vi "TCP Initialize Client.vi"   [LabVIEW 2016, in "SLL Easy API via TCP.lvclass"]
uses:
  SLL Easy API via TCP.lvclass
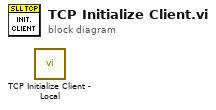
[diagram p0: block diagram]
diagram:
  n1 = call "TCP Initialize Client - Local.vi"() -> ()  [unwired: 10 in, 2 out]
